vi "RSZVB Initialize.vi"(6 "Serial Configuration":T1={"Baud Rate"=9600, "Flow Control"=0, "Parity"=0, "Data Bits"=7, "Stop Bits"=10} {"Stop Bits" items=["1.0"=10, "1.5"=15, "2.0"=20]; "Data Bits" items=["7"=7, "8"=8]; "Parity" items=["None", "Odd", "Even", "Mark", "Space"]; "Flow Control" items=["None"=0, "XON/XOFF"=1, "RTS/CTS"=2, "DTR/DSR"=4]; "Baud Rate" items=["300"=300, "600"=600, "1200"=1200, "2400"=2400, "4800"=4800, "9600"=9600, "19200"=19200]}, 8 "error in (no error)":errorcluster {"code" format="%.0x"}, 9 "Reset? (T: Yes)":bool=TRUE, 10 "ID Query? (T: Yes)":bool=TRUE, 11 "VISA Resource Name (GPIB::20)":refnum<visa-resource-name>) -> (0 "error out":errorcluster {"code" format="%.0x"}, 3 "dup VISA session":refnum<visa-resource-name>)   [LabVIEW 2015]
doc: "This VI passes the addressing information in the instrument decriptor to the Instr Open VI and returns the instrument ID. You can optionally reset the instrument by setting the front panel reset control. You must run this VI before using any of the instrument driver VIs for this instrument."
uses:
  _utility/RSZVB Global Data.vi
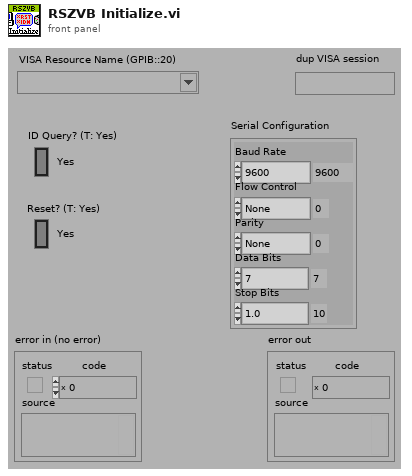
[diagram p1: front panel]
types:
  T1 = cluster{"Baud Rate":u32, "Flow Control":u16, "Parity":u16, "Data Bits":u16, "Stop Bits":u16}
  T2 = cluster{"Status":bool, "Code":i32, "Source (VI Name)":string}
  T3 = cluster{"Error Checking (T: On)":bool, "Installed Options":string[], "Data Valid?":bool, "Ports":i32, "Model":string[], "Error Checking (T: On) 2":bool}[]
  T4 = cluster{"Error Checking (T: On)":bool, "Installed Options":string[], "Data Valid?":bool, "Ports":i32, "Installed Options 2":string[], "Error Checking (T: On) 2":bool}[]
  T5 = cluster{"Error Checking (T: On)":bool, "Installed Options":string[], "Data Valid?":bool, "Ports":i32, "Model":string[], "Option Checking (T: On)":bool}[]
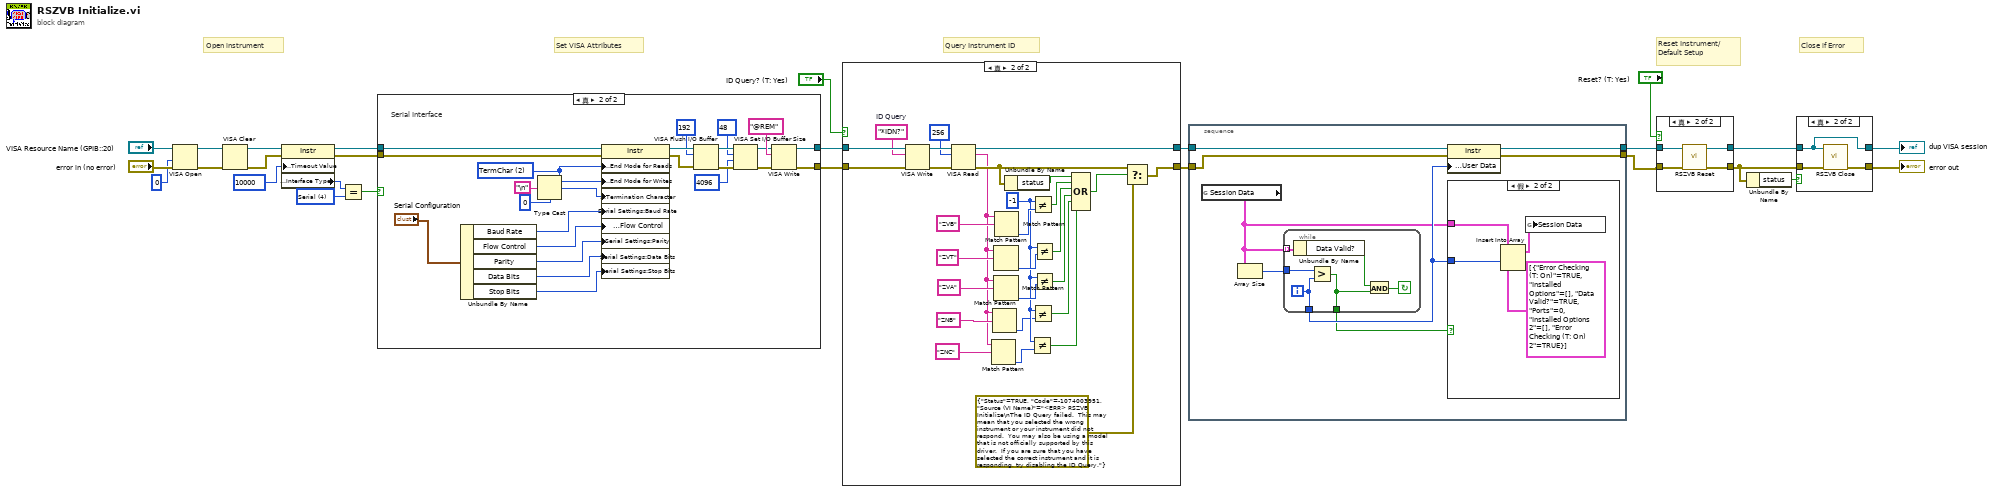
[diagram p0: block diagram]
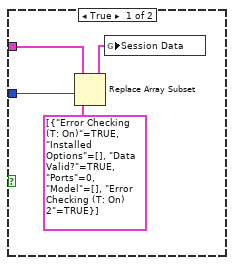
[diagram p2: hidden frame]
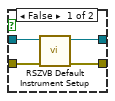
[diagram p5: hidden frame]
diagram:
  w12 = u16 4 items=["GPIB"=1, "VXI"=2, "GPIB-VXI"=3, "Serial"=4, "PXI"=5, "TCPIP"=6, "USB"=7] ("Interface Information:Interface Type")
  # "Set VISA Attributes"
  # "Close if Error"
  # "Query Instrument ID"
  # "Reset Instrument/\nDefault Setup"
  # "Open instrument"
  n1 = VISA Open(access mode=u32 0, error in (no error)="error in (no error)", VISA resource name="VISA Resource Name (GPIB::20)") -> (VISA resource name=w10:refnum<visa-resource-name>, error out=w9:errorcluster)  [unwired: 2 in]
  n2 = VISA Clear(VISA resource name=w10, error in (no error)=w9) -> (VISA resource name out=w8:refnum<visa-resource-name>, error out=w7:errorcluster)
  n3 = property class="Instr"(reference=w8, error in=w7, "General Settings:Timeout Value"=u32 10000) -> (reference out=w15:refnum<visa-resource-name>, error out=w14:errorcluster, "Interface Information:Interface Type"=w19:u16)
  n4 = Equal?(x=w19, y=w12) -> (x = y?=w13:bool)
  n5 = case shown="真" w13 {
    tunnel: [w27 w29] -> w17
    tunnel: [w28 w30] -> w16
    tunnel: w15 -> [w27 w51]
    tunnel: w14 -> [w28 w52]
    frame False {
      # "GPIB, TCP/IP, and USB Interface"
    }
    frame True {
      w41 = u16 2 items=["None", "LastBit", "TermChar"] ("Serial Settings:Serial End Mode for Reads")
      # "Serial Interface"
      n6 = Unbundle By Name("Serial Configuration") -> ("Baud Rate"=w38:u32, "Flow Control"=w37:u16, "Parity"=w34:u16, "Data Bits"=w36:u16, "Stop Bits"=w35:u16)
      n7 = Type Cast(type=u8 0, x="\n" ("Line Feed Constant")) -> (*(type *) &x=w40:u8)
      n8 = property class="Instr"(reference=w51, error in=w52, "Serial Settings:End Mode for Reads"=w41, "Serial Settings:End Mode for Writes"=w41, "Message Based Settings:Termination Character"=w40, "Serial Settings:Baud Rate"=w38, "Serial Settings:Flow Control"=w37, "Serial Settings:Parity"=w34, "Serial Settings:Data Bits"=w36, "Serial Settings:Stop Bits"=w35) -> (reference out=w47:refnum<visa-resource-name>, error out=w49:errorcluster)
      n9 = VISA Flush I/O Buffer(VISA resource name=w47, mask (16)=u16 192, error in (no error)=w49) -> (VISA resource name out=w50:refnum<visa-resource-name>, error out=w48:errorcluster)
      n10 = VISA Set I/O Buffer Size(VISA resource name=w50, mask (16)=u16 48, size (4096)=u32 4096 ("size (0)"), error in (no error)=w48) -> (VISA resource name out=w32:refnum<visa-resource-name>, error out=w31:errorcluster)
      n11 = VISA Write(VISA resource name=w32, write buffer="@REM" ("write buffer (\"\")"), error in (no error)=w31) -> (VISA resource name out=w29:refnum<visa-resource-name>, error out=w30:errorcluster)  [unwired: 1 out]
    }
  }
  n12 = case shown="真" "ID Query? (T: Yes)" {
    tunnel: [w53 w83] -> w4
    tunnel: [w54 w80] -> w3
    tunnel: w17 -> [w54 w81]
    tunnel: w16 -> [w53 w82]
    frame False {
    }
    frame True {
      w70 = "*IDN?"  # ID Query
      w60 = -1
      n13 = VISA Write(VISA resource name=w81, write buffer=w70, error in (no error)=w82) -> (VISA resource name out=w78:refnum<visa-resource-name>, error out=w76:errorcluster)  [unwired: 1 out]
      n14 = VISA Read(VISA resource name=w78, byte count=u32 256, error in (no error)=w76) -> (VISA resource name out=w80:refnum<visa-resource-name>, read buffer=w55:string, error out=w77:errorcluster)  [unwired: 1 out]
      n15 = Match Pattern(string=w55, regular expression="ZNC") -> (offset past match=w59:i32)  [unwired: 1 in, 3 out]
      n16 = Match Pattern(string=w55, regular expression="ZNB") -> (offset past match=w58:i32)  [unwired: 1 in, 3 out]
      n17 = Match Pattern(string=w55, regular expression="ZVT") -> (offset past match=w67:i32)  [unwired: 1 in, 3 out]
      n18 = Match Pattern(string=w55, regular expression="ZVA") -> (offset past match=w64:i32)  [unwired: 1 in, 3 out]
      n19 = Match Pattern(string=w55, regular expression="ZVB") -> (offset past match=w72:i32)  [unwired: 1 in, 3 out]
      n20 = Unbundle By Name(w77) -> ("status"=w74:bool)
      n21 = Not Equal?(x=w60, y=w59) -> (x != y?=w56:bool)
      n22 = Not Equal?(x=w60, y=w72) -> (x != y?=w79:bool)
      n23 = Not Equal?(x=w60, y=w58) -> (x != y?=w57:bool)
      n24 = Not Equal?(x=w60, y=w67) -> (x != y?=w66:bool)
      n25 = Not Equal?(x=w60, y=w64) -> (x != y?=w63:bool)
      n26 = Compound Arithmetic op=OR(w74, w79, w66, w63, w57, w56) -> (w75:bool)
      n27 = Select(t=w77, s=w75, f=T2 {"Status"=TRUE, "Code"=-1074003951, "Source (VI Name)"="<ERR> RSZVB Initialize\nThe ID Query failed.  This may mean that you selected the wrong instrument or your instrument did not respond.  You may also be using a model that is not officially supported by this driver.  If you are sure that you have selected the correct instrument and it is responding, try disabling the ID Query."}) -> (s? t:f=w83:T2)
    }
  }
  n28 = stacked-sequence {
    tunnel: w3 -> [w90]
    tunnel: w4 -> [w89]
    tunnel: [w87] -> w1
    tunnel: [w86] -> w2
    frame #0 {
      n29 = global read "RSZVB Global Data.vi" "Session Data"() -> (w84:T5)
      n30 = Array Size(array=w84) -> (size(s)=w91:i32)
      n31 = while {
        tunnel: w84 -> [w101] mode=indexing
        tunnel: w91 -> [w105]
        tunnel: [w104] -> w88
        tunnel: [w102] -> w85
        i -> [w104]
        stop <- w103 continue-if-true
        n32 = Unbundle By Name(w101) -> ("Data Valid?"=w100:bool)
        n33 = Greater?(x=w105, y=w104) -> (0:w102:bool)
        n34 = And(x=w100, y=w102) -> (x .and. y?=w103:bool)
      }
      n35 = property class="Instr"(reference=w90, error in=w89, "General Settings:User Data"=w88) -> (reference out=w87:refnum<visa-resource-name>, error out=w86:errorcluster)
      n36 = case shown="假" w85 {
        tunnel: w84 -> [w95 w99]
        tunnel: w88 -> [w94 w98]
        frame True {
          n37 = Replace Array Subset(array=w95, new element=T3 [{"Error Checking (T: On)"=TRUE, "Installed Options"=[], "Data Valid?"=TRUE, "Ports"=0, "Model"=[], "Error Checking (T: On) 2"=TRUE}] ("Session Data"), index=w94) -> (w93:T5)
          n38 = global write "RSZVB Global Data.vi" "Session Data"(w93) -> ()
        }
        frame False {
          n39 = Insert Into Array(array=w99, index=w98, new element=T4 [{"Error Checking (T: On)"=TRUE, "Installed Options"=[], "Data Valid?"=TRUE, "Ports"=0, "Installed Options 2"=[], "Error Checking (T: On) 2"=TRUE}] ("Session Data")) -> (w96:T5)
          n40 = global write "RSZVB Global Data.vi" "Session Data"(w96) -> ()
        }
      }
    }
  }
  n41 = case shown="真" "Reset? (T: Yes)" {
    tunnel: w2 -> [w109 w111]
    tunnel: [w108 w113] -> w6
    tunnel: [w107 w112] -> w24
    tunnel: w1 -> [w106 w110]
    frame False {
      n42 = call "RSZVB Default Instrument Setup.vi"("error in (no error)"=w109, "VISA session"=w106) -> ("error out"=w108:errorcluster, "dup VISA session"=w107:refnum<visa-resource-name>)  [unwired: 8 in]
    }
    frame True {
      n43 = call "RSZVB Reset.vi"("error in (no error)"=w111, "VISA session"=w110) -> ("error out"=w113:errorcluster, "dup VISA session"=w112:refnum<visa-resource-name>)  [unwired: 8 in]
    }
  }
  n44 = Unbundle By Name(w6) -> ("status"=w5:bool)
  n45 = case shown="真" w5 {
    tunnel: w24 -> [w115 w117]
    tunnel: [w115 w117] -> w23
    tunnel: [w114 w118] -> w22
    tunnel: w6 -> [w114 w116]
    frame False {
    }
    frame True {
      n46 = call "RSZVB Close.vi"("error in (no error)"=w116, "VISA session"=w117) -> ("error out"=w118:errorcluster)  [unwired: 9 in]
    }
  }
  "dup VISA session" <- w23
  "error out" <- w22
